vi "Kaelus PFE Preset.vi"(7 "Kaelus PFE":T2, 8 "error in (no error)":errorcluster, 11 "DAQmx Dev Name (FEModule)":string) -> (0 "error out":errorcluster, 3 "DAQmx Dev Name (FEModule)":string, 5 "PFE Position":T1)   [LabVIEW 2011]
uses:
  TypeDefs/Kaelus PFE Instrument Info.ctl
  BPIMCore EXT/HW IO/PIM Parameters.ctl
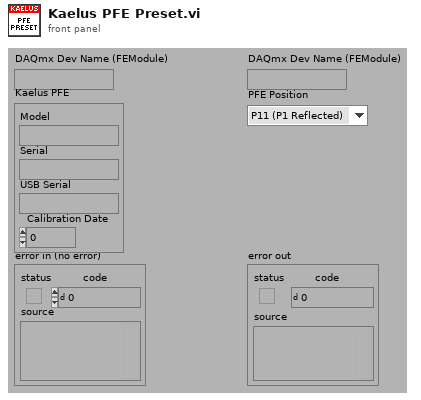
[diagram p1: front panel]
types:
  T1 = typedef "PIM Parameters.ctl" = enum16{"P11 (P1 Reflected)", "P12 (P2 Through)", "P21 (P1 Through)", "P22 (P2 Reflected)"}
  T2 = typedef "Kaelus PFE Instrument Info.ctl" = cluster{"Model":string, "Serial":string, "USB Serial":string, "Calibration Date":dbl}
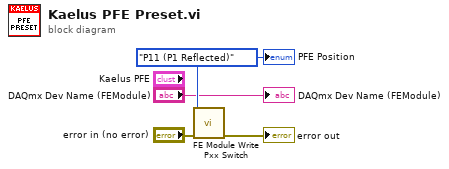
[diagram p0: block diagram]
diagram:
  w2 = PIM_Parameters."P11 (P1 Reflected)" ("Switch Position")
  n1 = call "FE Module Write Pxx Switch.vi"("error in (no error)"="error in (no error)", "P-Parameter"=w2) -> ("error out"=→"error out":errorcluster)  [unwired: 6 in]
  "DAQmx Dev Name (FEModule)" <- "DAQmx Dev Name (FEModule)"
  "PFE Position" <- w2
